vi "Configure Tag Current Pulse.vi"   [LabVIEW 2017, in "Keithley 2600 Series.lvlib"]
doc: "Configures a pulsed current sweep with a voltage measurement."
uses:
  <instrlib>/Keithley 2600 Series/Keithley 2600 Series.lvlib
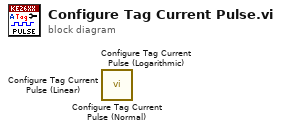
[diagram p0: block diagram]
diagram:
  n1 = call <instrlib>:"Configure Tag Current Pulse (Normal).vi"() -> ()  [unwired: 26 in, 2 out]
  n2 = call <instrlib>:"Configure Tag Current Pulse (Logarithmic).vi"() -> ()  [unwired: 26 in, 2 out]
  n3 = call <instrlib>:"Configure Tag Current Pulse (Linear).vi"() -> ()  [unwired: 26 in, 2 out]
